vi "6-1 hp34401.VI"() -> ()   [LabVIEW 2012]
panel:
  out "tensione":dbl
  in  "String":string="0.15"
  out "num string":dbl format="%.8f"
  out "Stringa di tensione":string
  # "Configurazione del multimetro (conf:volt:ac)  e  lettura  del dato (:read?)"
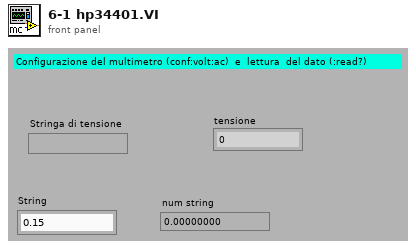
[diagram p1: front panel]
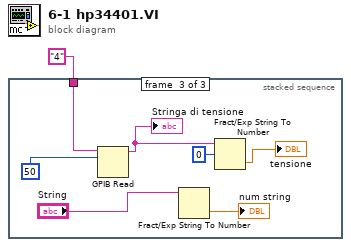
[diagram p0: block diagram]
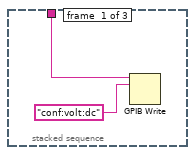
[diagram p2: hidden frame]
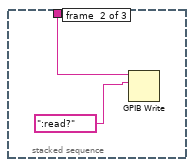
[diagram p3: hidden frame]
diagram:
  n1 = stacked-sequence {
    tunnel: "4" -> [w2 w4 w9]
    frame #0 {
      n2 = GPIB Write(0:w2, 1:"conf:volt:dc") -> ()  [unwired: 3 in, 2 out]
    }
    frame #1 {
      n3 = GPIB Write(0:w4, 1:":read?") -> ()  [unwired: 3 in, 2 out]
    }
    frame #2 {
      n4 = GPIB Read(0:w9, 1:50) -> (5:w8:string)  [unwired: 3 in, 2 out]
      "Stringa di tensione" <- w8
      n5 = Fract/Exp String To Number(string="String") -> (number=→"num string":dbl)  [unwired: 3 in, 1 out]
      n6 = Fract/Exp String To Number(string=w8, offset=0) -> (number=→"tensione":dbl)  [unwired: 2 in, 1 out]
    }
  }
